vi "PDE_Inject.vi"(11 "Rate":dbl=0.75) -> (3 "Number of samples":dbl)   [LabVIEW 2017]
uses:
  <vilib>/DAQmx/write.llb/DAQmx Write.vi
  <vilib>/DAQmx/write.llb/DAQmx Write (Digital 1D Wfm NChan NSamp).vi
  <vilib>/DAQmx/create/channels.llb/DAQmx Create Channel (DO-Digital Output).vi
  <vilib>/DAQmx/configure/timing.llb/DAQmx Timing (Sample Clock).vi
  <vilib>/Waveform/DWDTOps.llb/DWDT Uncompress Digital.vi
  <vilib>/DAQmx/miscellaneous.llb/DAQmx Fill In Error Info.vi
  <resource>/objmgr/daqmx.rc
panel:
  in  "error in":errorcluster
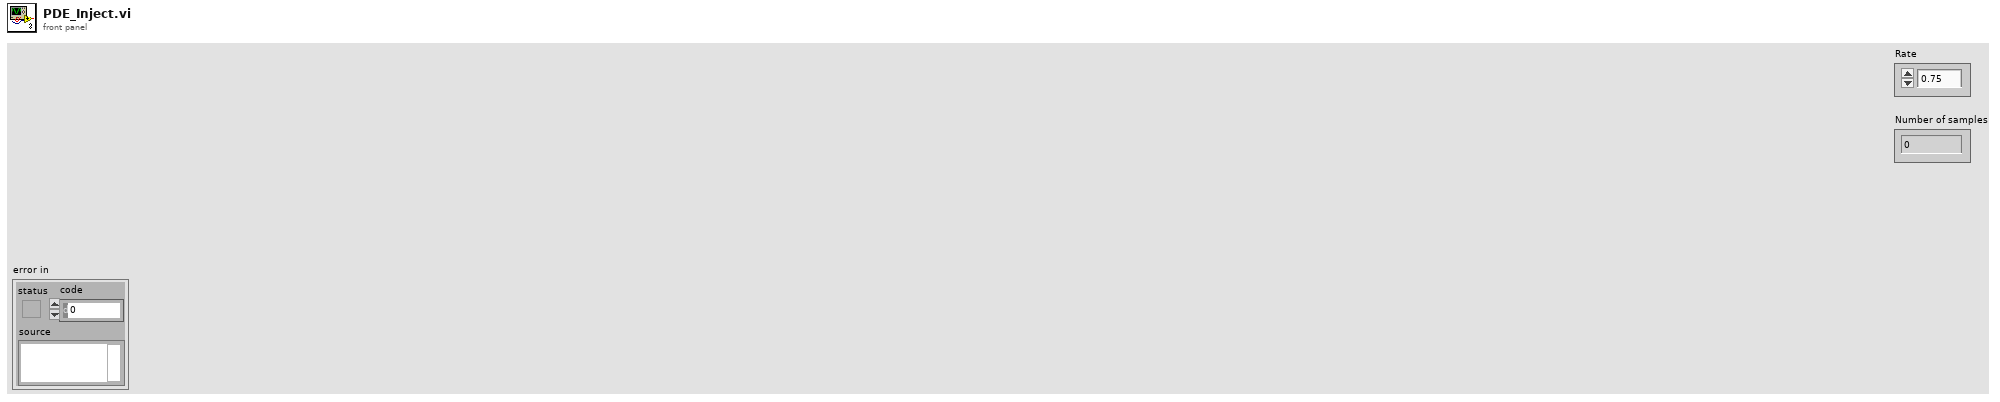
[diagram p1: front panel]
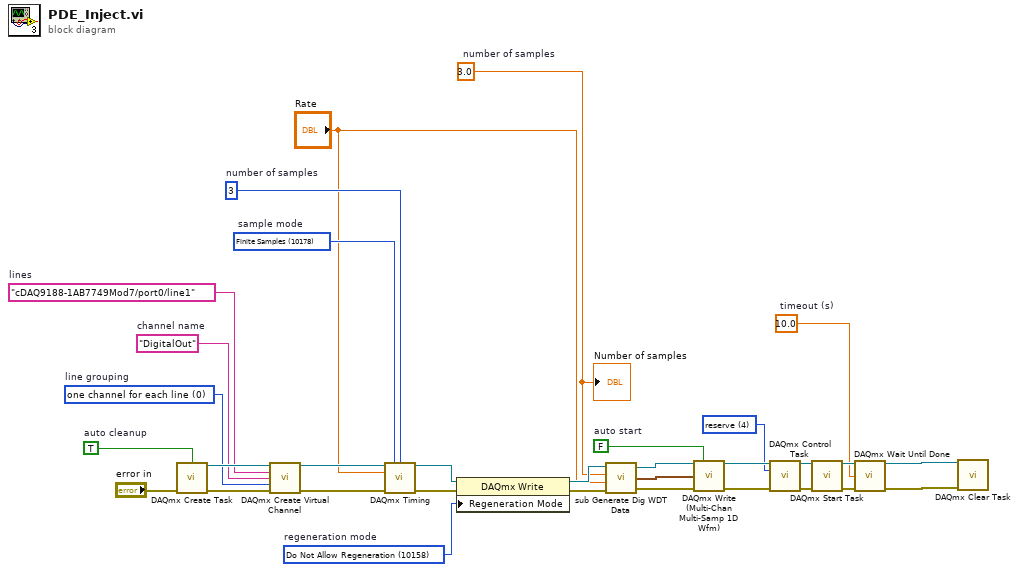
[diagram p0: block diagram]
diagram:
  w8 = 4 items=["verify"=2, "reserve"=4, "commit"=3, "unreserve"=5, "abort"=6] ("action")
  w2 = 10.0  # timeout (s)
  w13 = 10158 items=["Allow Regeneration"=10097, "Do Not Allow Regeneration"=10158]  # regeneration mode
  w15 = 10178 items=["Finite Samples"=10178, "Continuous Samples"=10123, "Hardware Timed Single Point"=12522]  # sample mode
  w16 = 3  # number of samples
  w21 = 0 items=["one channel for each line", "one channel for all lines"]  # line grouping
  w20 = "DigitalOut"  # channel name
  w22 = "cDAQ9188-1AB7749Mod7/port0/line1"  # lines
  w24 = TRUE  # auto cleanup
  w9 = 3.0  # number of samples
  w27 = FALSE  # auto start
  n1 = call <vilib>:"DAQmx Create Task.vi"("auto cleanup"=w24, "error in"="error in") -> ("task out"=w23:refnum<k21>, "error out"=w25:errorcluster)  [unwired: 12 in]
  n2 = call-poly <vilib>:"DAQmx Create Virtual Channel.vi"("task in"=w23, "lines"=w22, "name to assign"=w20, "line grouping"=w21, "error in"=w25) -> ("task out"=w17:refnum<k21>, "error out"=w19:errorcluster)  [unwired: 9 in]
  n3 = call-poly <vilib>:"DAQmx Timing.vi"("task/channels in"=w17, "sample mode"=w15, "samples per channel"=w16, "rate"="Rate", "error in"=w19) -> ("task out"=w14:refnum<k21>, "error out"=w18:errorcluster)  [unwired: 9 in]
  n4 = property class="DAQmx Write"(reference=w14, error in=w18, "Regeneration Mode"=w13) -> (reference out=w12:refnum<k21>, error out=w11:errorcluster)
  n5 = call <vilib>:"sub Generate Dig WDT Data.vi"("task in"=w12, "number of samples"=w9, "update rate"="Rate", "error in"=w11) -> ("task out"=w29:refnum<k21>, "data"=w30:digitalwaveform[], "error out"=w28:errorcluster)  [unwired: 1 in]
  n6 = call-poly "DAQmx Write (Multi-Chan Multi-Samp 1D Wfm).vi"("task/channels in"=w29, "auto start"=w27, "data"=w30, "error in"=w28) -> ("task out"=w32:refnum<k21>, "error out"=w31:errorcluster)  [unwired: 9 in, 1 out]
  n7 = call <vilib>:"DAQmx Control Task.vi"("task/channels in"=w32, "action"=w8, "error in"=w31) -> ("task out"=w1:refnum<k21>, "error out"=w7:errorcluster)  [unwired: 11 in]
  n8 = call <vilib>:"DAQmx Start Task.vi"("task/channels in"=w1, "error in"=w7) -> ("task out"=w6:refnum<k21>, "error out"=w5:errorcluster)  [unwired: 12 in]
  n9 = call <vilib>:"DAQmx Wait Until Done.vi"("task/channels in"=w6, "timeout (sec)"=w2, "error in"=w5) -> ("task out"=w3:refnum<k21>, "error out"=w4:errorcluster)  [unwired: 11 in]
  n10 = call <vilib>:"DAQmx Clear Task.vi"("task in"=w3, "error in"=w4) -> ()  [unwired: 13 in, 1 out]
  "Number of samples" <- w9
